vi "Save Binary format.vi"(5 "action":string="Save", 8 "error in":errorcluster, 10 "file path (use dialog)":path, 11 "data in":sgl[](array[numeric])) -> (0 "error out":errorcluster)   [LabVIEW 2018]
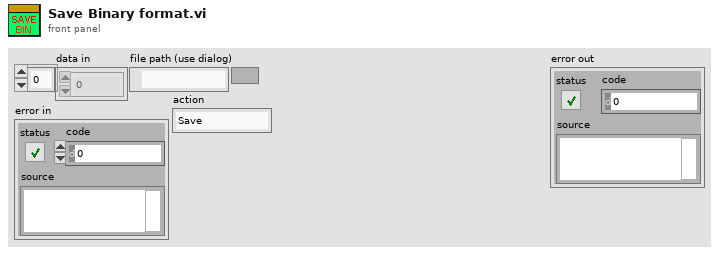
[diagram p1: front panel]
types:
  T1 = enum16{"big-endian, network order", "native, host order", "little-endian"}
  T2 = enum16{"open", "replace", "create", "open or create", "replace or create", "replace or create with confirmation"}
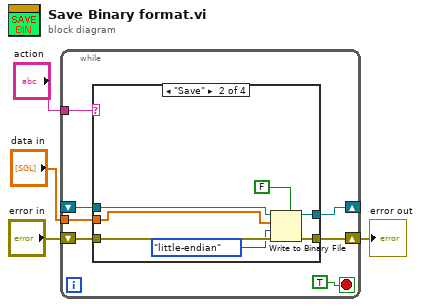
[diagram p0: block diagram]
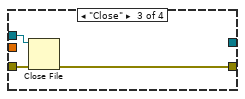
[diagram p3: hidden frame]
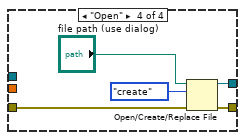
[diagram p4: hidden frame]
diagram:
  n1 = while {
    tunnel: "action" -> [w10]
    tunnel: "data in" -> [w9]
    shift-right: [w7] -> w1
    shift-left: "error in" -> [w8]
    shift-right: [w6] -> _
    shift-left: _ -> [w5]
    stop <- TRUE stop-if-true
    n2 = case shown="\"Save\"" w10 {
      tunnel: w9 -> [_ w20 _ _]
      tunnel: w8 -> [w13 w19 w23 w26]
      tunnel: [w13 w18 w21 w24] -> w7
      tunnel: [w12 w15 _ w28] -> w6
      tunnel: w5 -> [w12 w16 w22 _]
      frame "False", Default {
      }
      frame "Save" {
        n3 = Write to Binary File(file (use dialog)=w16, data=w20, error in=w19, 5:FALSE ("prepend array or string size? (T)"), 9:T1."little-endian" ("byte order (0:big-endian, network order)")) -> (refnum out=w15:refnum<file>, error out=w18:errorcluster)  [unwired: 1 in, 1 out]
      }
      frame "Close" {
        n4 = Close File(refnum=w22, error in=w23) -> (error out=w21:errorcluster)  [unwired: 1 out]
      }
      frame "Open" {
        n5 = Open/Create/Replace File(file path (use dialog)="file path (use dialog)", error in=w26, operation (0:open)=T2."create") -> (refnum out=w28:refnum<file>, error out=w24:errorcluster)  [unwired: 3 in, 1 out]
      }
    }
  }
  "error out" <- w1
